vi "cmdMotor.vi"(1 "Mode":enum16{"Position", "Velocity", "Torque"}(ring), 2 "Control Value":fxp<+/-,32,16>, 3 "ID":u32 format="%x", 4 "SPI Config In":T1) -> (0 "SPI Config Out":T1)   [LabVIEW 2019]
uses:
  SPI/SPI Config.ctl
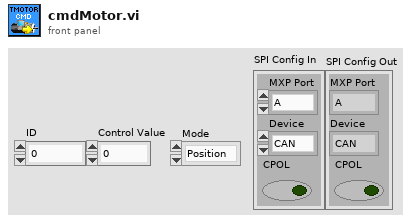
[diagram p1: front panel]
types:
  T1 = typedef "SPI Config.ctl" = cluster{"MXP Port":enum16{"A", "B"}, "Device":enum16{"CAN", "ENC", "IMU1", "IMU2"}, "CPOL":bool}
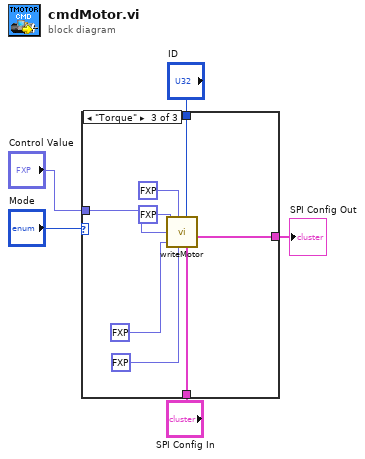
[diagram p0: block diagram]
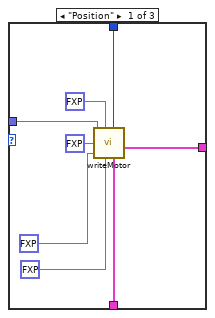
[diagram p2: hidden frame]
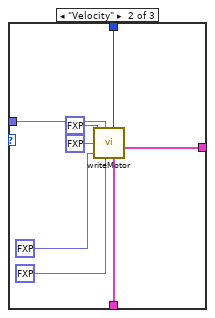
[diagram p3: hidden frame]
diagram:
  n1 = case shown="\"Torque\"" "Mode" {
    tunnel: [w13 w21 w29] -> w5
    tunnel: "ID" -> [w12 w20 w28]
    tunnel: "SPI Config In" -> [w11 w19 w27]
    tunnel: "Control Value" -> [w8 w17 w24]
    frame "Position" {
      n2 = call "writeMotor.vi"("Position"=w8, "Velocity"=fxp<+/-,32,16> 0.0, "Torque"=fxp<+/-,32,16> 0.0, "Kp"=fxp<+/-,32,16> 1.0, "Kd"=fxp<+/-,32,16> 1.0, "ID"=w12, "SPI Config In"=w11) -> ("SPI Config Out"=w13:T1)  [unwired: 3 in]
    }
    frame "Velocity" {
      n3 = call "writeMotor.vi"("Position"=fxp<+/-,32,16> 0.0, "Velocity"=w17, "Torque"=fxp<+/-,32,16> 0.0, "Kp"=fxp<+/-,32,16> 0.0, "Kd"=fxp<+/-,32,16> 1.0, "ID"=w20, "SPI Config In"=w19) -> ("SPI Config Out"=w21:T1)  [unwired: 3 in]
    }
    frame "Torque" {
      n4 = call "writeMotor.vi"("Position"=fxp<+/-,32,16> 0.0, "Velocity"=fxp<+/-,32,16> 0.0, "Torque"=w24, "Kp"=fxp<+/-,32,16> 0.0, "Kd"=fxp<+/-,32,16> 0.0 ("Kp"), "ID"=w28, "SPI Config In"=w27) -> ("SPI Config Out"=w29:T1)  [unwired: 3 in]
    }
  }
  "SPI Config Out" <- w5
